vi "FRC-Traj-Lib-analog-rate-limit-test-2.vi"() -> ()   [LabVIEW 2019]
uses:
  <vilib>/Rock Robotics/WPI/ThirdParty/JAS_Junk/TrajLib/Trajectory_Library.lvlib
panel:
  in  "Tab Control":enum32{"Control Panel", "Logic"}(tab)
  in  "Rate Limit":dbl=10.0
  in  "Input":dbl(slide)=10.0 scale=-100.0..100.0
  out "Output":dbl
  in  "Enable":bool
  out "Trend":cluster{"Input":dbl, "Output":dbl}(graph)
  out "Enabled":bool
  # "Rate Limit Test"
  # "Rate Limited"
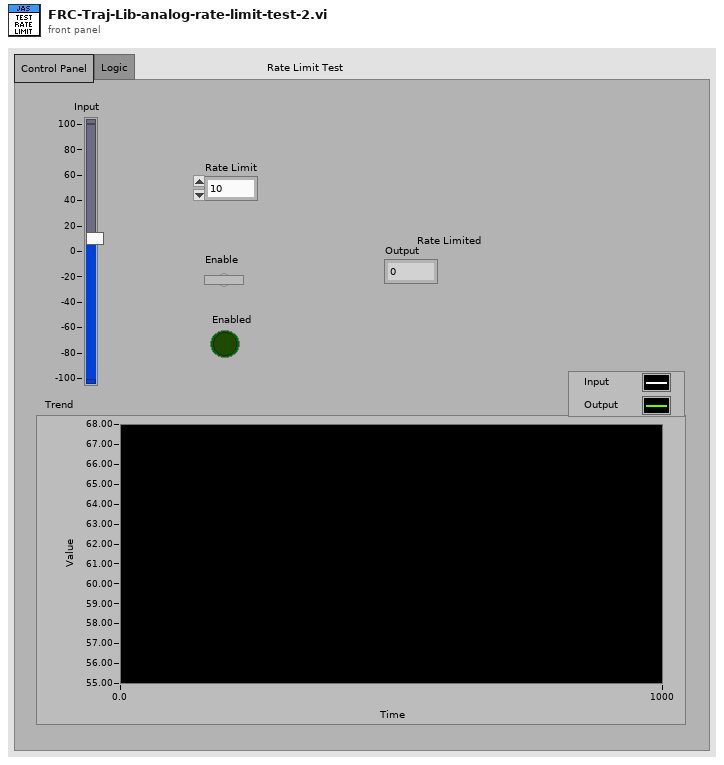
[diagram p1: front panel]
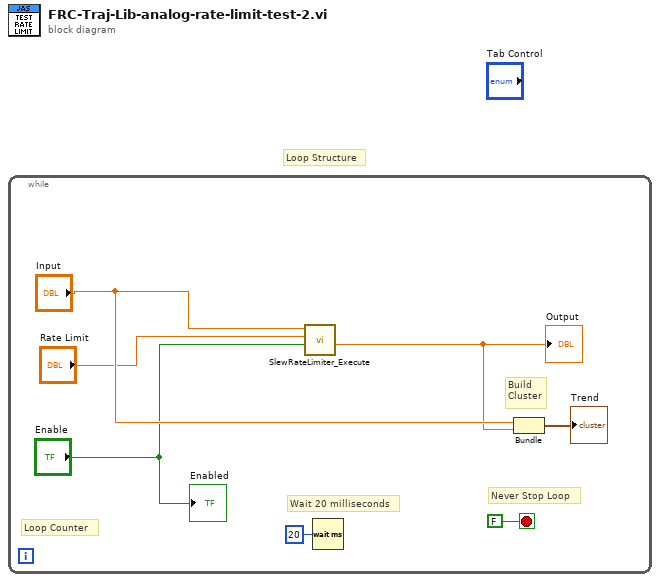
[diagram p0: block diagram]
diagram:
  # "Loop Structure"
  n1 = while {
    stop <- FALSE stop-if-true
    # "Build\nCluster"
    # "Loop Counter"
    # "Never Stop Loop"
    # "Wait 20 milliseconds"
    n2 = call <vilib>:"SlewRateLimiter_Execute.vi"("Enable"="Enable", "Rate"="Rate Limit", "Input"="Input") -> ("Output"=w1:dbl)  [unwired: 7 in, 1 out]
    "Output" <- w1
    n3 = Wait (ms)(milliseconds to wait=u32 20) -> ()  [unwired: 1 out]
    n4 = Bundle("Input"="Input", "Output"=w1) -> (→"Trend":cluster{"Input":dbl, "Output":dbl})  [unwired: 1 in]
    "Enabled" <- "Enable"
  }
